vi "GetMeasureFilterType.vi"(7 "SMU":T2, 8 "Error In":errorcluster, 11 "Kiethley 2602 In":refnum<visa-resource-name>) -> (0 "Error Out":errorcluster, 2 "Filter Type":T1, 3 "Keithley 2602 Out":refnum<visa-resource-name>)   [LabVIEW 2012, in "Keithley-2602.lvlib"]
uses:
  Keithley-2602.lvlib
  Controls/SMU.ctl
  Controls/FilterType.ctl
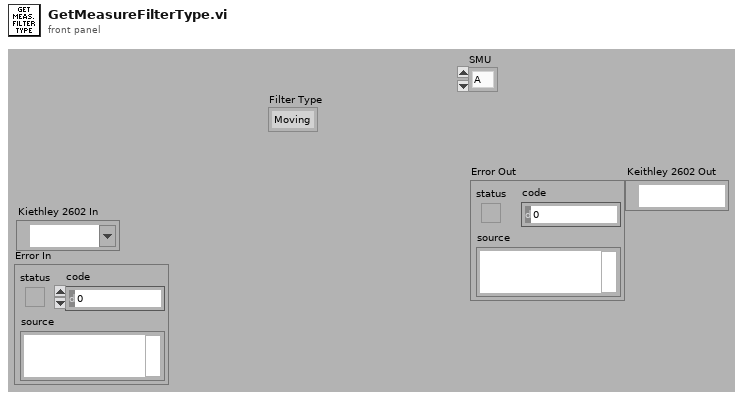
[diagram p1: front panel]
types:
  T1 = typedef "Keithley-2602.lvlib/FilterType.ctl" = enum16{"Moving", "Repeating", "Median"}
  T2 = typedef "Keithley-2602.lvlib/SMU.ctl" = enum16{"A", "B"}
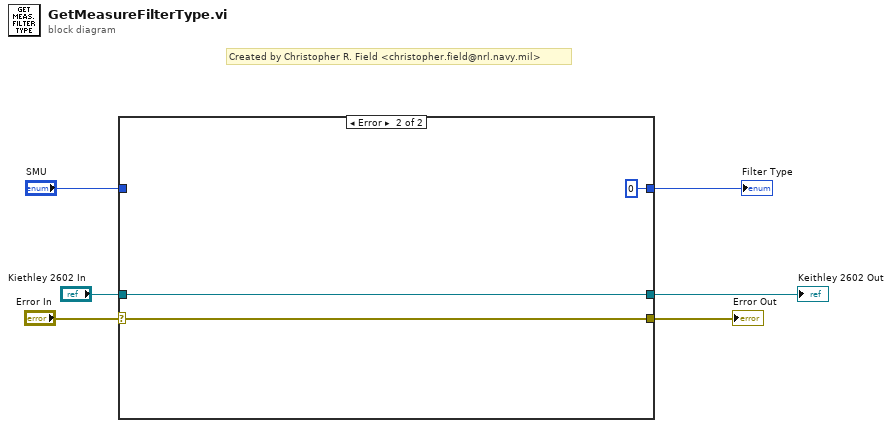
[diagram p0: block diagram]
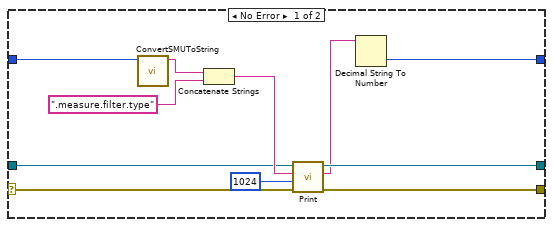
[diagram p2: hidden frame]
diagram:
  # "Created by Christopher R. Field <christopher.field@nrl.navy.mil>"
  n1 = case shown="Error" "Error In" {
    selector: "Error In" -> [w7 w20]
    tunnel: "Kiethley 2602 In" -> [w13 w19]
    tunnel: [w12 w20] -> w5
    tunnel: [w11 w19] -> w4
    tunnel: "SMU" -> [w9 _]
    tunnel: [w8 0] -> w2
    frame No Error {
      n2 = call "ConvertSMUToString.vi"("SMU"=w9) -> ("Channel"=w17:string)  [unwired: 10 in]
      n3 = Concatenate Strings(w17, ".measure.filter.type") -> (w15:string)
      n4 = call "Print.vi"("Error In"=w7, "Byte Count"=u32 1024, "Attribute"=w15, "Kiethley 2602 In"=w13) -> ("Error Out"=w12:errorcluster, "Output"=w10:string, "Keithley 2602 Out"=w11:refnum<visa-resource-name>)  [unwired: 5 in]
      n5 = Decimal String To Number(string=w10) -> (number=w8:i32)  [unwired: 2 in, 1 out]
    }
    frame Error {
    }
  }
  "Error Out" <- w5
  "Keithley 2602 Out" <- w4
  "Filter Type" <- w2
